vi "Set Arm (Enum).vi"(8 "error in (no error)":errorcluster, 11 "Arm":enum16{"Down", "Up"}(ring)) -> (0 "error out":errorcluster)   [LabVIEW 2011]
uses:
  Apendage State.ctl
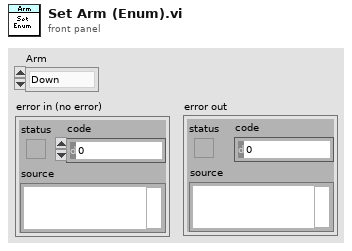
[diagram p1: front panel]
types:
  T1 = typedef "Apendage State.ctl" = enum16{"Unknown", "Down", "Up"}
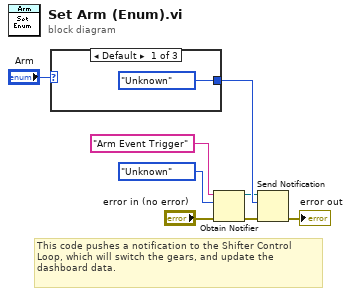
[diagram p0: block diagram]
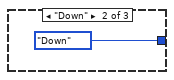
[diagram p2: hidden frame]
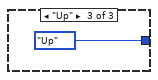
[diagram p3: hidden frame]
diagram:
  # "This code pushes a notification to the Shifter Control Loop, which will switch the gears, and update the dashboard data."
  n1 = case shown="Default" "Arm" {
    tunnel: [Apendage_State."Unknown" Apendage_State."Down" Apendage_State."Up"] -> w7
    frame Default {
    }
    frame "Down" {
    }
    frame "Up" {
    }
  }
  n2 = Obtain Notifier(name (unnamed)="Arm Event Trigger", notification data type=Apendage_State."Unknown", error in (no error)="error in (no error)") -> (notifier out=w4:refnum<notifier>, error out=w5:errorcluster)  [unwired: 1 in, 1 out]
  n3 = Send Notification(notification=w7, notifier=w4, error in (no error)=w5) -> (error out=→"error out":errorcluster)  [unwired: 1 out]
